vi "Open Tree.vi"(8 "error in (no error)":errorcluster, 9 "Shot":i32, 10 "Tree":string, 11 "Connection in":refnum<class "Connection.lvclass">) -> (0 "error out":errorcluster, 3 "Connection out":refnum<class "Connection.lvclass">)   [LabVIEW 2012, in "MDSplus.lvlib" / "Connection.lvclass"]
uses:
  <vilib>/MDSplus/Classes/Connection_Class/Connection.lvclass
  <vilib>/MDSplus/Classes/Connection_Class/Connection.lvclass/Connection.ctl
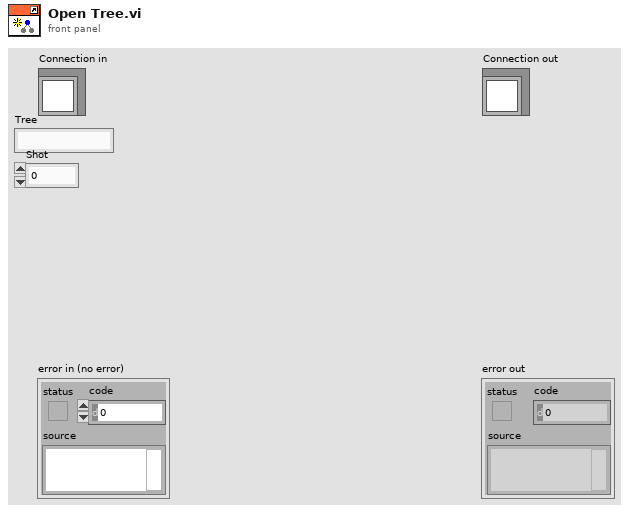
[diagram p1: front panel]
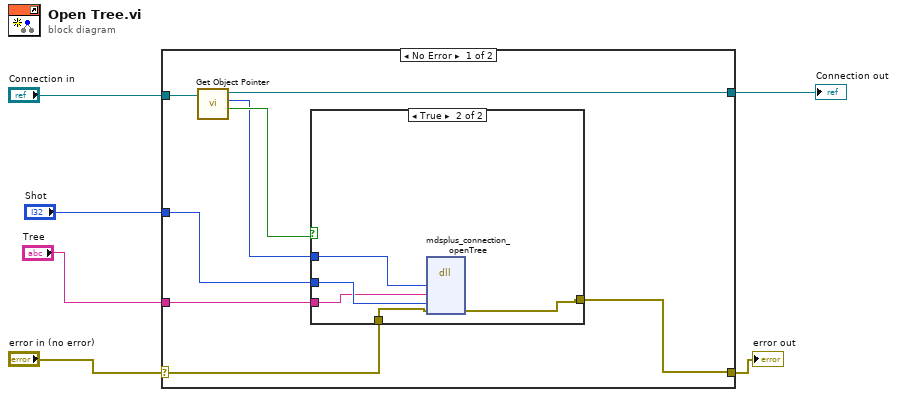
[diagram p0: block diagram]
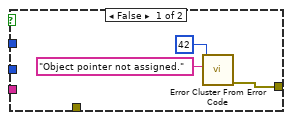
[diagram p2: hidden frame]
diagram:
  n1 = case shown="No Error" "error in (no error)" {
    selector: "error in (no error)" -> [w9 w24]
    tunnel: [w7 w24] -> w5
    tunnel: [w11 w23] -> w3
    tunnel: "Connection in" -> [w12 w23]
    tunnel: "Shot" -> [w10 _]
    tunnel: "Tree" -> [w8 _]
    frame No Error {
      n2 = call <vilib>:"Get Object Pointer.vi"("Connection in"=w12) -> ("Assigned object pointer?"=w14:bool, "Object Pointer"=w13:i64, "Connection out"=w11:refnum<class "Connection.lvclass">)  [unwired: 7 in, 1 out]
      n3 = case shown="True" w14 {
        tunnel: [w15 w18] -> w7
        tunnel: w13 -> [_ w22]
        tunnel: w10 -> [_ w20]
        tunnel: w9 -> [_ w21]
        tunnel: w8 -> [_ w19]
        frame False {
          n4 = call <vilib>:"Error Cluster From Error Code.vi"("error message (\"\")"="Object pointer not assigned." ("error message (\"\")"), "error code (0)"=42) -> ("error out"=w15:errorcluster)  [unwired: 7 in]
        }
        frame True {
          n5 = dll-call lib="MDSobjectsLVShr" fn="mdsplus_connection_openTree"("lvConnection"=w22, "treeIn"=w19, "shotIn"=w20, "error"=w21) -> ("error"=w18:errorcluster)  [unwired: 7 in, 2 out]
        }
      }
    }
    frame Error {
    }
  }
  "error out" <- w5
  "Connection out" <- w3
